vi "Write to CSV.vi"() -> ()   [LabVIEW 2019]
uses:
  <vilib>/Utility/file.llb/Write Delimited Spreadsheet (string).vi
  <vilib>/Utility/file.llb/Write Delimited Spreadsheet (DBL).vi
panel:
  in  "Number of Channels":dbl
  in  "Values to Generate":dbl
  in  "Channel Names":string[](array[string])
  in  "Header Info":string[][](array[string])
  in  "File Name":path
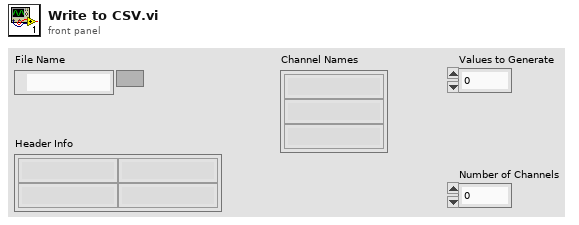
[diagram p1: front panel]
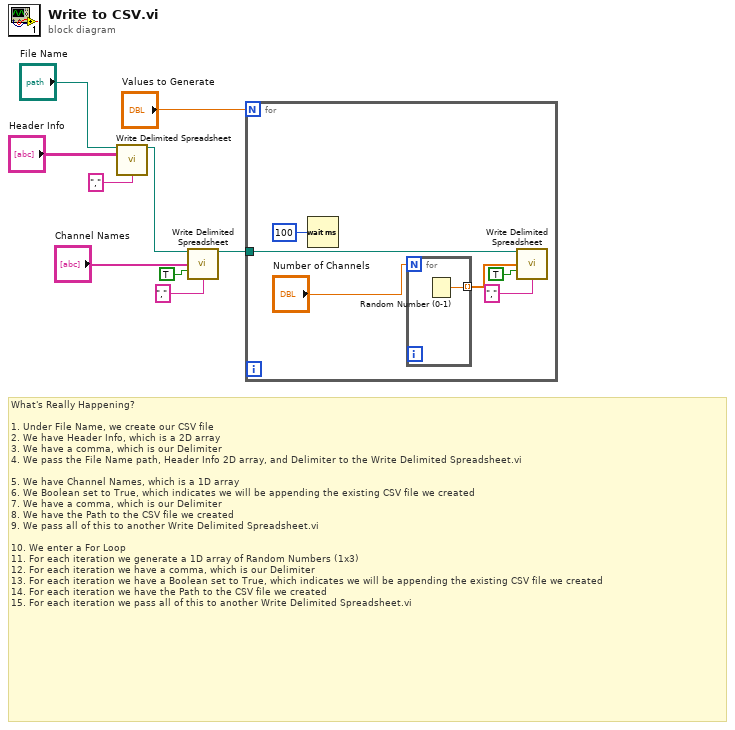
[diagram p0: block diagram]
diagram:
  # "What's Really Happening?\n\n1. Under File Name, we create our CSV file\n2. We have Header Info, which is a 2D array\n3. We have a comma, which is our Delimiter\n4. We pass the File Name path, Header Info 2D array, and Delimiter to the Write Delimited Spreadsheet.vi\n\n5. We have Channel Names, which is a 1D array\n6. We Boolean set to True, which indicates we will be appending the existing CSV file we created\n7. We have a comma, which is our Delimiter\n8. We have the Path to the CSV file we created\n9. We pass all of this to another Write Delimited Spreadsheet.vi\n\n10. We enter a For Loop\n11. For each iteration we generate a 1D array of Random Numbers (1x3)\n12. For each iteration we have a comma, which is our Delimiter\n13. For each iteration we have a Boolean set to True, which indicates we will be appending the existing CSV file we created\n14. For each iteration we have the Path to the CSV file we created\n15. For each iteration we pass all of this to another Write Delimited Spreadsheet.vi"
  n1 = call-poly <vilib>:"Write Delimited Spreadsheet.vi"("file path (dialog if empty)"="File Name", "2D data"="Header Info", "delimiter (\\t)"=",") -> ("new file path (Not A Path if cancelled)"=w6:path)  [unwired: 11 in, 1 out]
  n2 = call-poly <vilib>:"Write Delimited Spreadsheet.vi"("file path (dialog if empty)"=w6, "1D data"="Channel Names", "append to file? (new file:F)"=TRUE, "delimiter (\\t)"=",") -> ("new file path (Not A Path if cancelled)"=w1:path)  [unwired: 10 in, 1 out]
  n3 = for {
    N: "Values to Generate" -> [_]
    tunnel: w1 -> [w11]
    n4 = Wait (ms)(milliseconds to wait=100) -> ()  [unwired: 1 out]
    n5 = for {
      N: "Number of Channels" -> [_]
      tunnel: [w16] -> w12 mode=indexing
      n6 = Random Number (0-1)() -> (number: 0 to 1=w16:dbl)
    }
    n7 = call-poly <vilib>:"Write Delimited Spreadsheet.vi"("file path (dialog if empty)"=w11, "1D data"=w12, "append to file? (new file:F)"=TRUE, "delimiter (\\t)"=",") -> ()  [unwired: 10 in, 2 out]
  }
